vi "RichToFlatnixnet_grpc_ReadSignalXYResponse.vi"(5 "OutputClusterType":T1, 11 "InputCluster":T2) -> (3 "OutputCluster":T1)   [LabVIEW 2025, in "xnet-grpc_client.lvlib"]
uses:
  nixnet_grpc_ReadSignalXYResponse.ctl
  nixnet_grpc_ReadSignalXYResponse_Flat.ctl
  xnet-grpc_client.lvlib
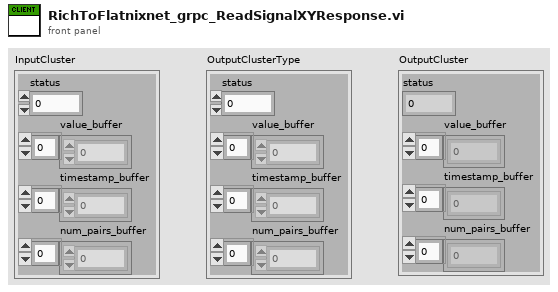
[diagram p1: front panel]
types:
  T1 = typedef "xnet-grpc_client.lvlib/nixnet_grpc_ReadSignalXYResponse_Flat.ctl" = cluster{"status":i32, "value_buffer":dbl[], "timestamp_buffer":u64[], "num_pairs_buffer":u32[]}
  T2 = typedef "xnet-grpc_client.lvlib/nixnet_grpc_ReadSignalXYResponse.ctl" = cluster{"status":i32, "value_buffer":dbl[], "timestamp_buffer":u64[], "num_pairs_buffer":u32[]}
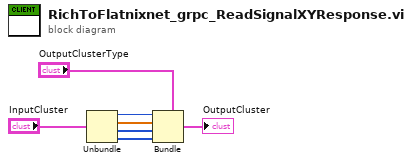
[diagram p0: block diagram]
diagram:
  n1 = Unbundle "Unbundle"("InputCluster") -> ("status"=w4:i32, "value_buffer"=w3:dbl[], "timestamp_buffer"=w2:u64[], "num_pairs_buffer"=w1:u32[])
  n2 = Bundle "Bundle"(cluster="OutputClusterType", "status"=w4, "value_buffer"=w3, "timestamp_buffer"=w2, "num_pairs_buffer"=w1) -> (→"OutputCluster":T1)
